vi "niFpgaDdsAccum.vi"(8 "init":bool, 9 "frequency_scaled":fxp<+,32,0>) -> (1 "new_period":bool, 2 "current_accum_state":fxp<+,32,0> format="%.32g")   [LabVIEW 2017]
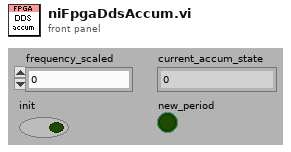
[diagram p1: front panel]
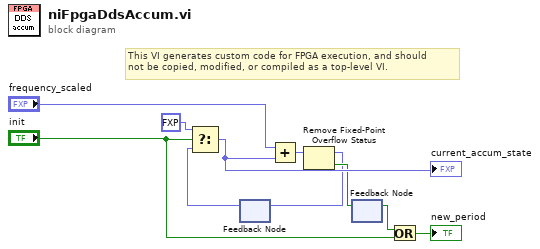
[diagram p0: block diagram]
diagram:
  # "This VI generates custom code for FPGA execution, and should\nnot be copied, modified, or compiled as a top-level VI."
  n1 = feedback #1() -> (w7:fxp<+,32,0>)  [unwired: 1 out]
  n2 = Select(t=fxp<+,32,0> 0.0, s="init", f=w7) -> (s? t:f=w4:fxp<+,32,0>)
  "current_accum_state" <- w4
  n3 = Add(x="frequency_scaled", y=w4) -> (x+y=w3:fxp<+,32,0>)
  n4 = Remove Fixed-Point Overflow Status(3:w3) -> (0:w2:bool, 1:w1:fxp<+,32,0>)
  n5 = feedback-in #1(w1) -> ()
  n6 = feedback-in #2(w2) -> ()
  n7 = feedback #2() -> (w5:bool)  [unwired: 1 out]
  n8 = Or(x=w5, y="init") -> (x .or. y?=→"new_period":bool)
